vi "MGCC_FntStaMach_voltagedifference_figureplot.vi"(1 "array":cdb[][](array[numeric]), 2 "index (row)":i32) -> (0 "output cluster":cluster{dbl[], dbl[]})   [LabVIEW 2016]
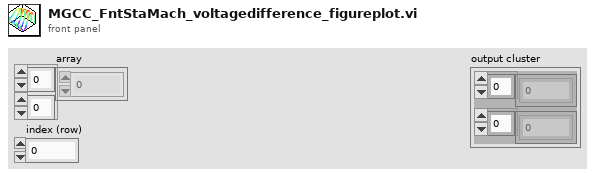
[diagram p1: front panel]
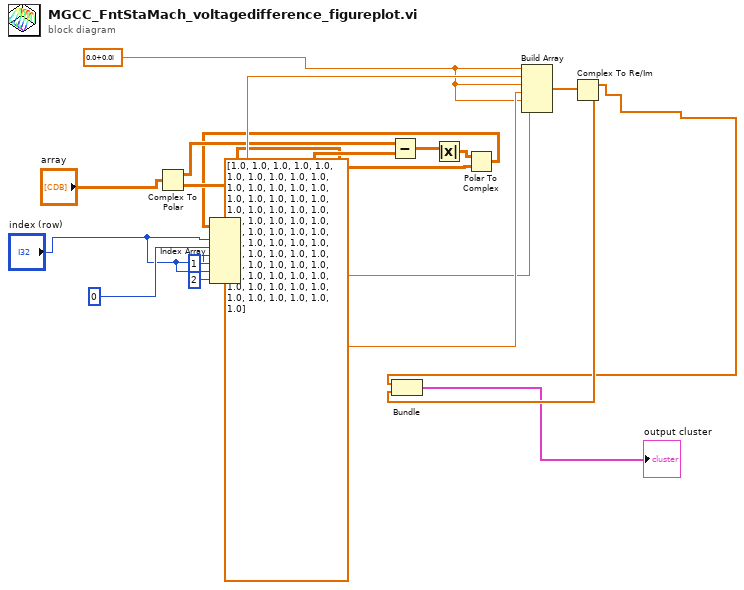
[diagram p0: block diagram]
diagram:
  w11 = csg 0.0+0.0i ("element")
  n1 = Complex To Polar(r * e^(i*theta)="array") -> (r=w7:dbl[][], theta=w2:dbl[][])
  n2 = Subtract(x=w7, y=dbl[][] [[1.0, 1.0, 1.0], [1.0, 1.0, 1.0], [1.0, 1.0, 1.0], [1.0, 1.0, 1.0], [1.0, 1.0, 1.0], [1.0, 1.0, 1.0], [1.0, 1.0, 1.0], [1.0, 1.0, 1.0], [1.0, 1.0, 1.0], [1.0, 1.0, 1.0], [1.0, 1.0, 1.0], [1.0, 1.0, 1.0], [1.0, 1.0, 1.0], [1.0, 1.0, 1.0], [1.0, 1.0, 1.0], [1.0, 1.0, 1.0], [1.0, 1.0, 1.0], [1.0, 1.0, 1.0], [1.0, 1.0, 1.0], [1.0, 1.0, 1.0], [1.0, 1.0, 1.0], [1.0, 1.0, 1.0]]) -> (x-y=w5:dbl[][])
  n3 = Absolute Value(x=w5) -> (abs(x)=w3:dbl[][])
  n4 = Polar To Complex(1:w2, 2:w3) -> (0:w1:cdb[][])
  n5 = Index Array(array=w1, index (row) #1="index (row)", index (col) #1=0 ("disabled index (col)"), index (row) #2="index (row)", index (col) #2=1 ("disabled index (col)"), index (row) #3="index (row)", index (col) #3=2 ("disabled index (col)")) -> (element #1=w15:cdb, element #2=w16:cdb, element #3=w14:cdb)
  n6 = Build Array(w11, w15, w11, w16, w11, w14) -> (w13:cdb[])
  n7 = Complex To Re/Im(x + iy=w13) -> (x=w4:dbl[], y=w12:dbl[])
  n8 = Bundle(w4, w12) -> (→"output cluster":cluster{dbl[], dbl[]})  [unwired: 1 in]
